vi "DHE_DRV_set_guide_mode.vi"(0 "fd":i32, 1 "exptime":i32, 7 "guide":bool, 11 "error in (no error)":errorcluster, 12 "rows":i32, 13 "cols":i32) -> (4 "fd out":i32, 8 "return value":i32, 15 "error out":errorcluster)   [LabVIEW 2016]
doc: "This VI closes the I/O interface with the instrument."
uses:
  c/lib/libarcDHE.so
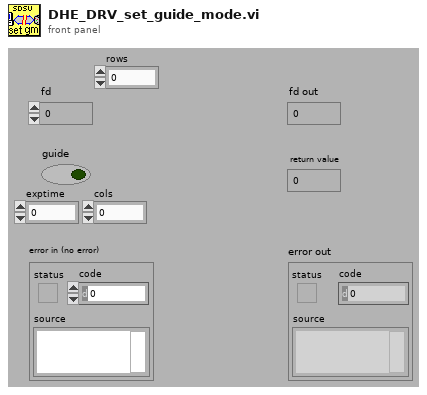
[diagram p1: front panel]
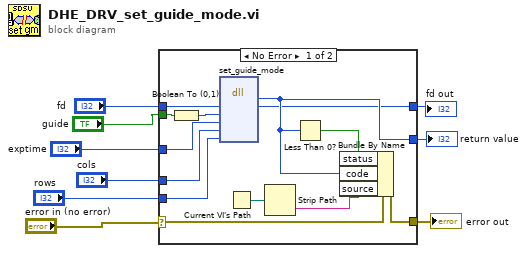
[diagram p0: block diagram]
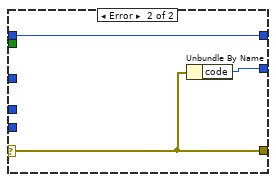
[diagram p2: hidden frame]
diagram:
  n1 = case shown="No Error" "error in (no error)" {
    selector: "error in (no error)" -> [w15 w24]
    tunnel: "fd" -> [w22 w25]
    tunnel: [w20 w23] -> w8
    tunnel: [w17 w24] -> w7
    tunnel: [w16 w25] -> w6
    tunnel: "guide" -> [w14 _]
    tunnel: "exptime" -> [w12 _]
    tunnel: "cols" -> [w11 _]
    tunnel: "rows" -> [w10 _]
    frame No Error {
      n2 = Boolean To (0,1)(Boolean=w14) -> (0, 1=w13:i16)
      n3 = dll-call lib="home/simager/panview/PAN/Modules/SDSU/private/c/lib/libarcDHE.so" fn="set_guide_mode"("fd"=w22, "gmode"=w13, "exptime"=w12, "cols"=w11, "rows"=w10) -> ("return type"=w20:i32, "fd"=w16:i32)  [unwired: 6 in, 3 out]
      n4 = Current VI's Path() -> (path=w19:path)
      n5 = Strip Path(path=w19) -> (name=w18:string)  [unwired: 1 out]
      n6 = Less Than 0?(x=w20) -> (x < 0?=w21:bool)
      n7 = Bundle By Name(cluster=w15, "status"=w21, "code"=w20, "source"=w18) -> (w17:errorcluster)
    }
    frame Error {
      n8 = Unbundle By Name(w24) -> ("code"=w23:i32)
    }
  }
  "error out" <- w7
  "return value" <- w8
  "fd out" <- w6
